vi "吸光值辅助计算.vi"() -> (2 "X":dbl format="%#.6f", 3 "吸光值导出":u16(ring) items=["不导入", "标样一", "标样二", "标样三", "零点", "跨度"])   [LabVIEW 2016, in "斯坦道总磷.lvlib"]
panel:
  in  "F3":dbl
  in  "F2":dbl
  in  "确认":bool
  in  "导入至":u16(ring) items=["不导入", "标样一", "标样二", "标样三", "零点", "跨度"]
  in  "F1":dbl
  in  "F0":dbl
  in  "吸光值算法":enum16{"氨氮、总磷、营养盐、CODcr", "氨氮-OPA", "总氮、COD"}(ring)
  # "吸光值辅助计算"
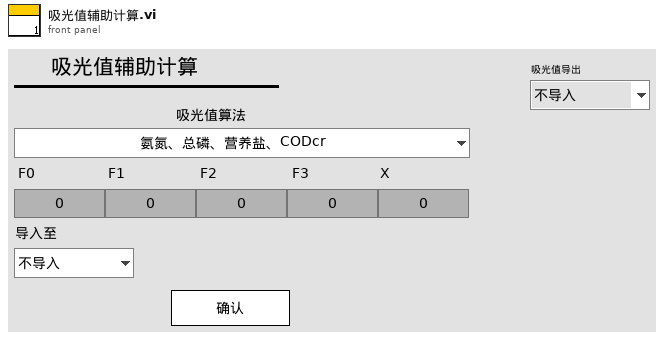
[diagram p1: front panel]
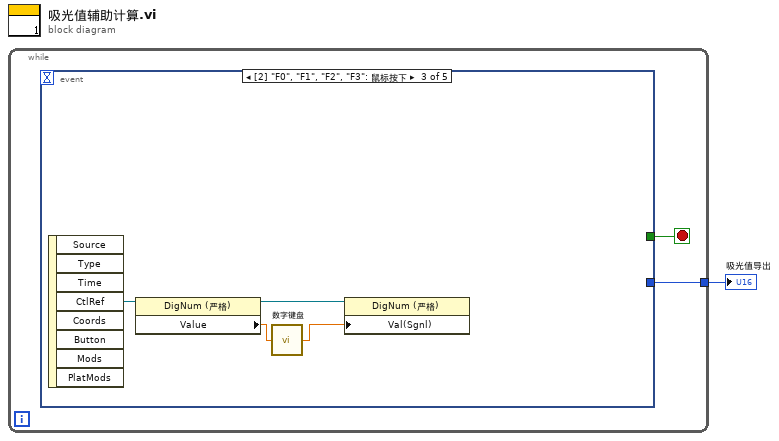
[diagram p0: block diagram]
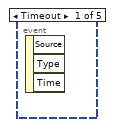
[diagram p2: hidden frame]
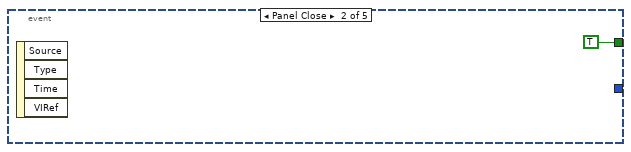
[diagram p3: hidden frame]
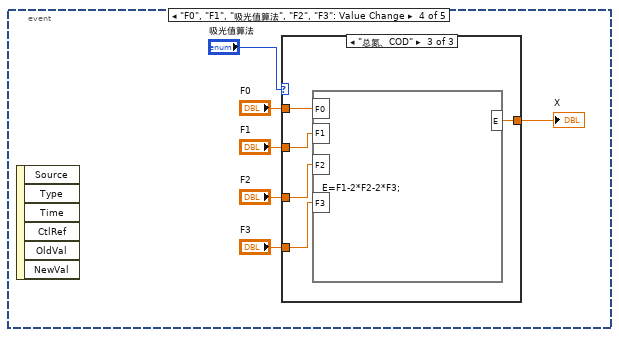
[diagram p4: hidden frame]
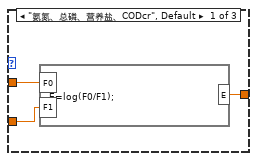
[diagram p5: hidden frame]
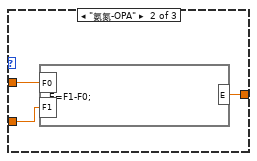
[diagram p6: hidden frame]
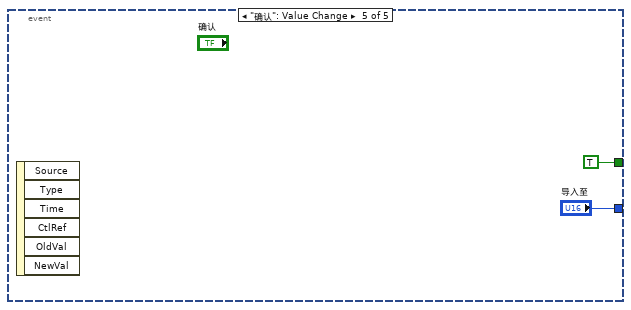
[diagram p7: hidden frame]
diagram:
  n1 = while {
    tunnel: [w2] -> w1
    stop <- w3 stop-if-true
    n2 = event shown="[2] \"F0\", \"F1\", \"F2\", \"F3\": 鼠标按下" {
      selector: _ -> [_ _ _ _ _]
      dyn-events: _ -> [_ _ _ _ _]
      timeout: _ -> [_ _ _ _ _]
      tunnel: [_ TRUE _ _ TRUE] -> w3
      tunnel: [_ _ _ _ "导入至"] -> w2
      event Timeout {
        n3 = event-data() -> ()  [unwired: 1 in, 3 out]
      }
      event Panel Close {
        n4 = event-data() -> ()  [unwired: 1 in, 4 out]
      }
      event "F0", "F1", "F2", "F3": Mouse Down {
        n5 = event-data() -> ("CtlRef"=w8:refnum<vi>)  [unwired: 1 in, 7 out]
        n6 = property class="DigNum (严格)"(reference=w8) -> (reference out=w5:refnum<vi>, "Value"=w7:dbl)  [unwired: 1 in, 1 out]
        n7 = call "数字键盘.vi"("OldNumber"=w7) -> ("NewNumber"=w6:dbl)
        n8 = property class="DigNum (严格)"(reference=w5, "Val(Sgnl)"=w6) -> ()  [unwired: 1 in, 2 out]
      }
      event "F0", "F1", "吸光值算法", "F2", "F3": Value Change {
        n9 = event-data() -> ()  [unwired: 1 in, 6 out]
        n10 = case shown="\"总氮、COD\"" "吸光值算法" {
          tunnel: "F0" -> [w17 w20 w25]
          tunnel: "F1" -> [w16 w19 w24]
          tunnel: [w15 w18 w23] -> w14
          tunnel: "F2" -> [_ _ w22]
          tunnel: "F3" -> [_ _ w21]
          frame "氨氮、总磷、营养盐、CODcr", Default {
            n11 = formula code="E=log(F0/F1);"("F0"=w17, "F1"=w16) -> ("E"=w15:dbl)
          }
          frame "氨氮-OPA" {
            n12 = formula code="E=F1-F0;"("F0"=w20, "F1"=w19) -> ("E"=w18:dbl)
          }
          frame "总氮、COD" {
            n13 = formula code="E=F1-2*F2-2*F3;"("F0"=w25, "F1"=w24, "F2"=w22, "F3"=w21) -> ("E"=w23:dbl)
          }
        }
        "X" <- w14
      }
      event "确认": Value Change {
        n14 = event-data() -> ()  [unwired: 1 in, 6 out]
      }
    }
  }
  "吸光值导出" <- w1
